vi "Read Build Name.vi"(8 "error in (no error)":errorcluster, 11 "Build Job in":refnum<class "Build Job.lvclass">) -> (0 "error out":errorcluster, 2 "Build Name":string, 3 "Build Job out":refnum<class "Build Job.lvclass">)   [LabVIEW 2014, in "Build Job.lvclass"]
uses:
  Build Job.lvclass
  Build Job.lvclass/Build Job.ctl
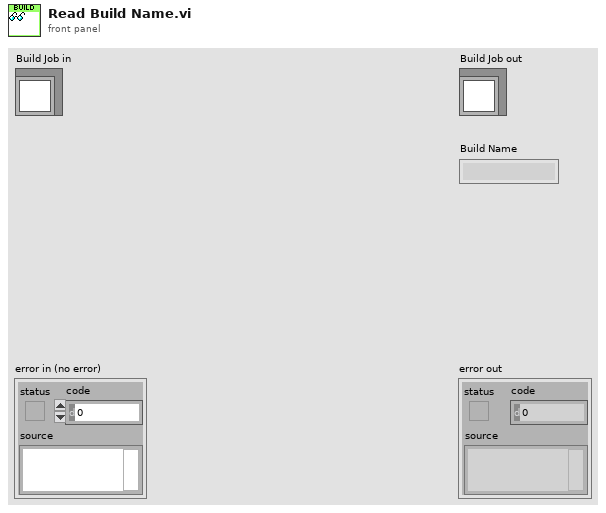
[diagram p1: front panel]
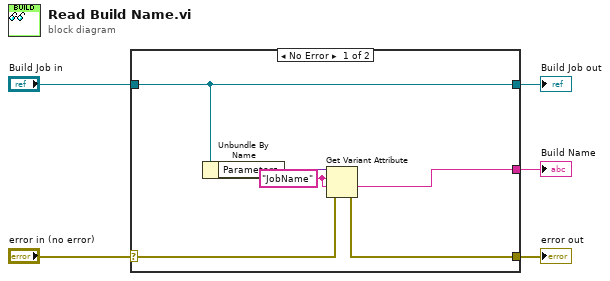
[diagram p0: block diagram]
diagram:
  n1 = case shown="No Error" "error in (no error)" {
    selector: "error in (no error)" -> [w7 w12]
    tunnel: [w6 w12] -> w4
    tunnel: [w11 w13] -> w2
    tunnel: "Build Job in" -> [w11 w13]
    tunnel: [w8 _] -> w1
    frame No Error {
      w9 = "JobName" ("name")
      n2 = Unbundle By Name(w11) -> ("Parameters"=w10:variant)
      n3 = Get Variant Attribute(Variant=w10, name=w9, default value (empty Variant)=w9, error in=w7) -> (value=w8:string, error out=w6:errorcluster)  [unwired: 2 out]
    }
    frame Error {
    }
  }
  "error out" <- w4
  "Build Job out" <- w2
  "Build Name" <- w1
